vi "generare metrici.vi"() -> ()   [LabVIEW 2024]
uses:
  <vilib>/Utility/file.llb/Write Delimited Spreadsheet (I64).vi
  <vilib>/National Instruments/NI Super Simple Neural Networks/Neural Network.lvclass
panel:
  out "F1 Score":dbl
  out "Acuratete":dbl
  out "Matricea de confuzie":dbl[][](array[numeric])
  in  "Cale salvare matricea de confuzie":path
  in  "Model antrenat":path
  in  "Data folder":path
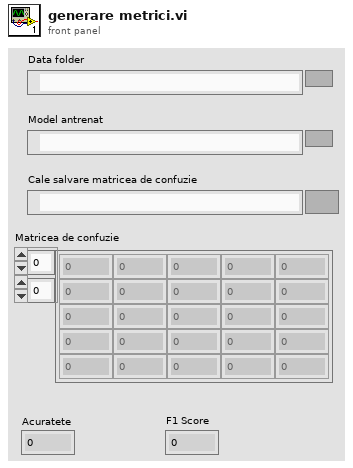
[diagram p1: front panel]
types:
  T1 = enum16{"Normalizare [0,1]", "Normalizare[-1,1]", "Fara normalizare"}
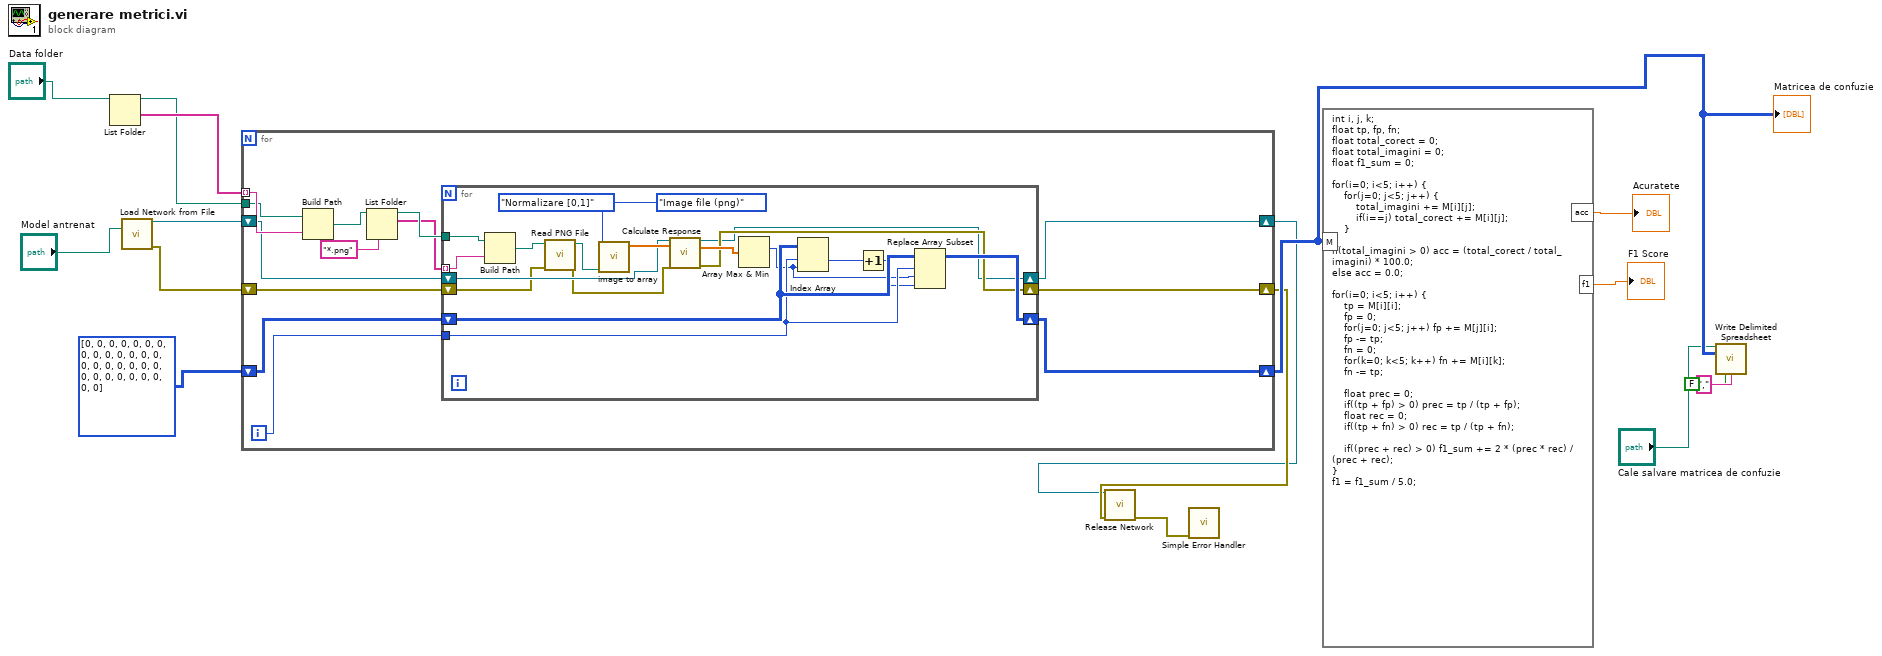
[diagram p0: block diagram]
diagram:
  n1 = List Folder(path="Data folder") -> (path out=w11:path, folder names=w14:string[])  [unwired: 3 in, 2 out]
  n2 = call <vilib>:"Load Network from File.vi"("File Path (dialog)"="Model antrenat") -> ("Neural Network Out"=w13:refnum<class "Neural Network.lvclass">, "Error Out"=w4:errorcluster)  [unwired: 11 in, 2 out]
  n3 = for {
    shift-right: [w20] -> w8
    shift-left: i32[][] [[0, 0, 0, 0, 0, 0], [0, 0, 0, 0, 0, 0], [0, 0, 0, 0, 0, 0], [0, 0, 0, 0, 0, 0], [0, 0, 0, 0, 0, 0]] -> [w23]
    tunnel: w14 -> [w29] mode=indexing
    tunnel: w11 -> [w24]
    shift-right: [w18] -> w3
    shift-left: w4 -> [w19]
    shift-right: [w17] -> w1
    shift-left: w13 -> [w21]
    i -> [w22]
    n4 = Build Path(base path=w24, name or relative path=w29) -> (appended path=w28:path)
    n5 = List Folder(path=w28, pattern="*.png") -> (path out=w26:path, filenames=w25:string[])  [unwired: 2 in, 2 out]
    n6 = for {
      tunnel: w26 -> [w48]
      tunnel: w25 -> [w47] mode=indexing
      tunnel: w22 -> [w39]
      shift-right: [w36] -> w20
      shift-left: w23 -> [w40]
      shift-right: [w33] -> w18
      shift-left: w19 -> [w35]
      shift-right: [w32] -> w17
      shift-left: w21 -> [w43]
      n7 = Build Path(base path=w48, name or relative path=w47) -> (appended path=w46:path)
      n8 = call <vilib>:"Read PNG File.vi"("error in (no error)"=w35, "path to PNG file"=w46) -> ("error out"=w34:errorcluster, "path"=w45:path)  [unwired: 7 in, 1 out]
      n9 = call "image to array.vi"("Path to PNG file"=w45, "Normalizare"=T1."Normalizare [0,1]", "Image type"=enum16{"Image file (png)", "Image data"}."Image file (png)") -> ("Image 1d Array"=w44:dbl[])  [unwired: 4 in, 4 out]
      n10 = call <vilib>:"Calculate Response.vi"("Neural Network In"=w43, "Inputs"=w44, "Error In"=w34) -> ("Neural Network Out"=w32:refnum<class "Neural Network.lvclass">, "Outputs"=w42:dbl[], "Error Out"=w33:errorcluster)  [unwired: 10 in]
      n11 = Array Max & Min(array=w42) -> (max index (indices)=w38:i32)  [unwired: 3 out]
      n12 = Index Array(array=w40, index (row)=w39, index (col)=w38) -> (element=w41:i32)
      n13 = Increment(x=w41) -> (x+1=w37:i32)
      n14 = Replace Array Subset(array=w40, new element=w37, index (row)=w39, index (col)=w38) -> (w36:i32[][])
    }
  }
  "Matricea de confuzie" <- w8
  n15 = call <vilib>:"Release Network.vi"("Neural Network"=w1, "Error In"=w3) -> ("Error Out"=w2:errorcluster)  [unwired: 13 in]
  n16 = call <vilib>:"Simple Error Handler.vi"("error in (no error)"=w2) -> ()  [unwired: 4 in, 5 out]
  n17 = formula code="int i, j, k;\nfloat tp, fp, fn;\nfloat total_corect = 0;\nfloat total_imagini = 0;\nfloat f1_sum = 0;\n\nfor(i=0; i<5; i++) {\n    for(j=0; j<5; j++) {\n        total_imagini += M[i][j];\n        if(i==j) total_corect += M[i][j];\n    }\n}\nif(total_imagini > 0) acc = (total_corect / total_imagini) * 100.0;\nelse acc = 0.0;\n\nfor(i=0; i<5; i++) {\n    tp = M[i][i]; \n    fp = 0; \n    for(j=0; j<5; j++) fp += M[j][i];\n    fp -= tp;\n    fn = 0;\n    for(k=0; k<5; k++) fn += M[i][k];\n    fn -= tp;\n    \n    float prec = 0;\n    if((tp + fp) > 0) prec = tp / (tp + fp);\n    float rec = 0;\n    if((tp + fn) > 0) rec = tp / (tp + fn);\n    \n    if((prec + rec) > 0) f1_sum += 2 * (prec * rec) / (prec + rec);\n}\nf1 = f1_sum / 5.0;"("M"=w8) -> ("acc"=→"Acuratete":dbl, "f1"=→"F1 Score":dbl)
  n18 = call-poly <vilib>:"Write Delimited Spreadsheet.vi"("file path (dialog if empty)"="Cale salvare matricea de confuzie", "2D data"=w8, "transpose? (no:F)"=FALSE, "delimiter (\\t)"="," ("delimiter (\\t)")) -> ()  [unwired: 10 in, 2 out]
